vi "Get Trigger Level Range.vi"(8 "error in (no error)":errorcluster, 10 "maximum":sgl, 11 "minimum":sgl) -> (0 "error out":errorcluster, 1 "function return":u32, 2 "maximum out":sgl, 3 "minimum out":sgl)   [LabVIEW 2014, in "atmcd32d.lvlib"]
doc: "unsigned int WINAPI GetTriggerLevelRange(float * minimum, float * maximum);"
uses:
  atmcd32d.lvlib
  atmcd32d.dll
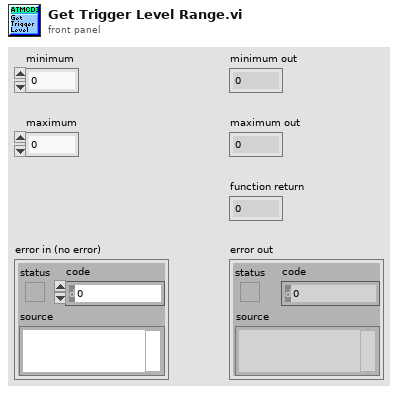
[diagram p1: front panel]
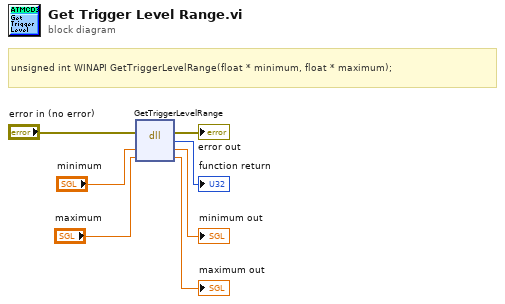
[diagram p0: block diagram]
diagram:
  # "unsigned int WINAPI GetTriggerLevelRange(float * minimum, float * maximum);"
  n1 = dll-call lib="C:/Users/Bakir/Documents/Lambda2-Testing/lib/Andorlib/atmcd32d.*" fn="GetTriggerLevelRange"(error in="error in (no error)", "minimum"="minimum", "maximum"="maximum") -> (error out=→"error out":errorcluster, →"function return":u32, "minimum"=→"minimum out":sgl, "maximum"=→"maximum out":sgl)  [unwired: 2 in, 1 out]
